vi "TopLeft Visible Cell Index.vi"(10 "Top Left Visible Cell":T2, 11 "TreeItems":T1[](array[typedef])) -> (3 "TreeItem idex (Top left visible)":i32)   [LabVIEW 2020, in "BetterDragAndDrop.lvlib" / "BetterTreeHandle.lvclass"]
uses:
  Classes/BetterTreeHandle/BetterTreeHandle.lvclass
  <vilib>/Utility/miscctls.llb/LVNodeAndColumnTypeDef.ctl
  Classes/BetterTreeItem/SubVIs/TreeItem.ctl
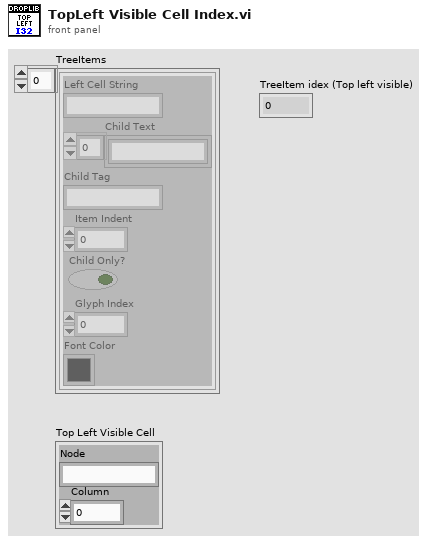
[diagram p1: front panel]
types:
  T1 = typedef "BetterDragAndDrop.lvlib/BetterTreeHandle.lvclass/TreeItem.ctl" = cluster{"Left Cell String":string, "Child Text":string[], "Child Tag":string, "Item Indent":i32, "Child Only?":bool, "Glyph Index":i32, "Font Color":u32}
  T2 = typedef "LVNodeAndColumnTypeDef.ctl" = cluster{"Node":string, "Column":i32}
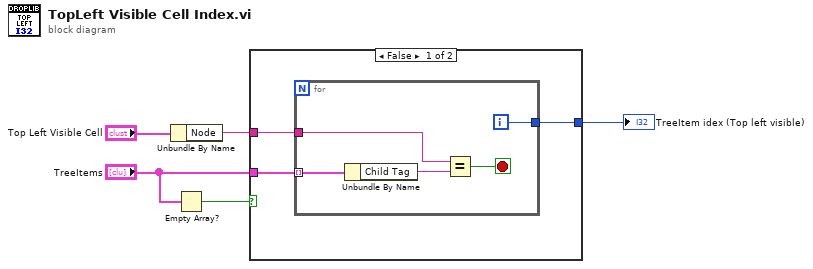
[diagram p0: block diagram]
diagram:
  n1 = Unbundle By Name("Top Left Visible Cell") -> ("Node"=w4:string)
  n2 = Empty Array?(array="TreeItems") -> (empty?=w1:bool)
  n3 = case shown="False" w1 {
    tunnel: w4 -> [w8 _]
    tunnel: "TreeItems" -> [w7 _]
    tunnel: [w6 _] -> w2
    frame False {
      n4 = for {
        tunnel: [w11] -> w6
        tunnel: w7 -> [w13] mode=indexing
        tunnel: w8 -> [w10]
        i -> [w11]
        stop <- w9 stop-if-true
        n5 = Unbundle By Name(w13) -> ("Child Tag"=w12:string)
        n6 = Equal?(x=w10, y=w12) -> (x = y?=w9:bool)
      }
    }
    frame True {
    }
  }
  "TreeItem idex (Top left visible)" <- w2
